vi "SecondaryJoystickButtonMapping.vi"(9 "Secondary joystick buttons":bool[](array[boolean])) -> (0 "Secondary joystick buttons indicator":bool[](array[boolean]), 3 "SecondaryJoystickButtons":T1)   [LabVIEW 2019]
uses:
  Controls/SecondaryJoystickButtons.ctl
panel:
  in  "SecondaryJoystickButtons 2":T1
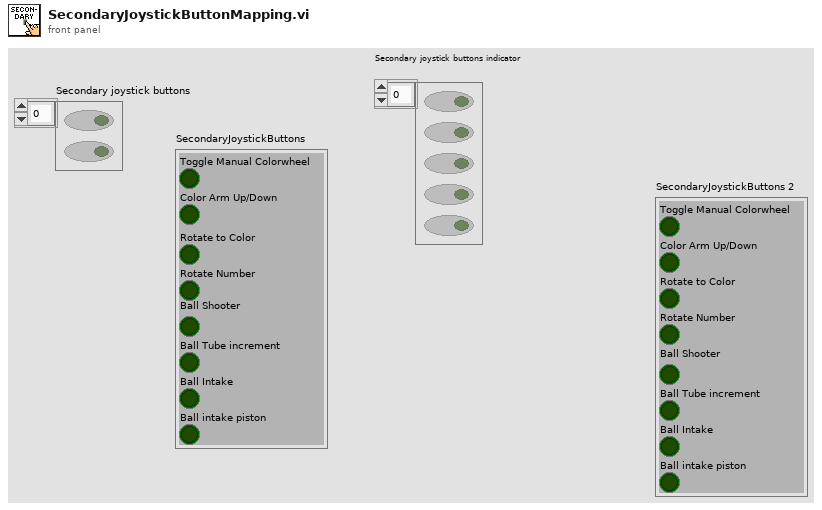
[diagram p1: front panel]
types:
  T1 = typedef "SecondaryJoystickButtons.ctl" = cluster{"Toggle Manual Colorwheel":bool, "Color Arm Up/Down":bool, "Rotate to Color":bool, "Rotate Number":bool, "Ball Shooter":bool, "Ball Tube increment":bool, "Ball Intake":bool, "Ball intake piston":bool}
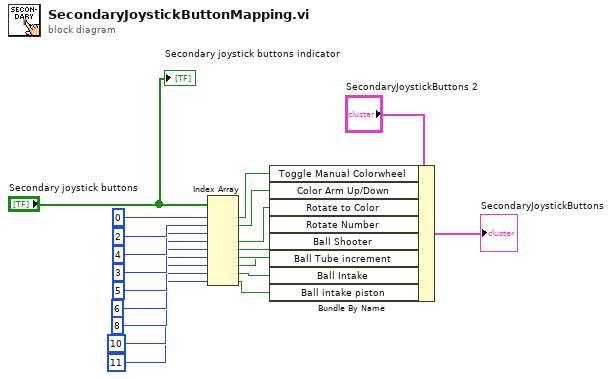
[diagram p0: block diagram]
diagram:
  n1 = Index Array(array="Secondary joystick buttons", index #1=0 ("index"), index #2=2 ("index"), index #3=4 ("index"), index #4=3 ("index"), index #5=5 ("index"), index #6=6 ("index"), index #7=8 ("index"), index #8=10 ("index"), index #9=11 ("index")) -> (element #1=w19:bool, element #2=w18:bool, element #4=w17:bool, element #5=w16:bool, element #6=w15:bool, element #7=w14:bool, element #8=w13:bool, element #9=w12:bool)  [unwired: 1 out]
  n2 = Bundle By Name(cluster="SecondaryJoystickButtons 2", "Toggle Manual Colorwheel"=w19, "Color Arm Up/Down"=w18, "Rotate to Color"=w17, "Rotate Number"=w16, "Ball Shooter"=w15, "Ball Tube increment"=w14, "Ball Intake"=w13, "Ball intake piston"=w12) -> (→"SecondaryJoystickButtons":T1)
  "Secondary joystick buttons indicator" <- "Secondary joystick buttons"
